vi "thermistor_manager_2.vi"(8 "ready for output (T)":bool=TRUE, 9 "input valid":bool=TRUE, 11 "indexed_voltage":T2) -> (3 "indexed_temperature":T1)   [LabVIEW 2018]
uses:
  indexed_analog.ctl
  indexed_fxp32_16.ctl
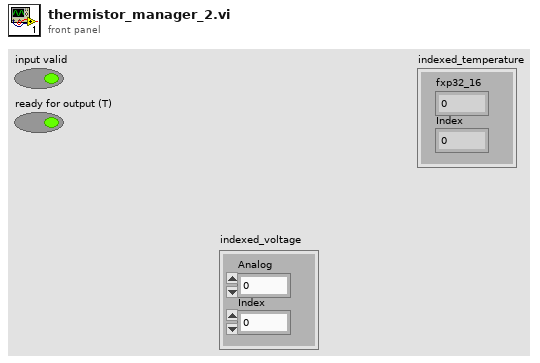
[diagram p1: front panel]
types:
  T1 = typedef "indexed_fxp32_16.ctl" = cluster{"fxp32_16":fxp<+/-,32,16>, "Index":fxp<+,3,3>}
  T2 = typedef "indexed_analog.ctl" = cluster{"Analog":fxp<+/-,24,5>, "Index":fxp<+,3,3>}
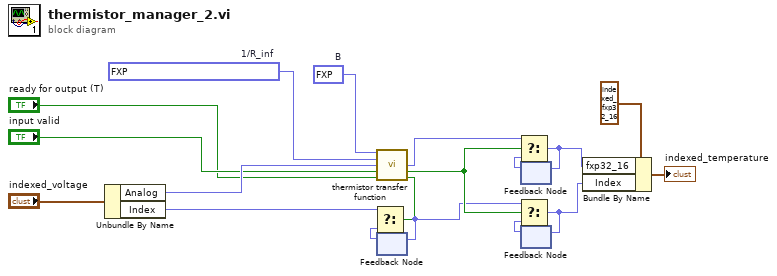
[diagram p0: block diagram]
diagram:
  w16 = fxp<+,32,7> 10.047783523797989  # 1/R_inf
  w17 = fxp<+/-,32,16> 3434.0  # B
  n1 = Unbundle By Name("indexed_voltage") -> ("Analog"=w14:fxp<+/-,24,5>, "Index"=w2:fxp<+,3,3>)
  n2 = call "thermistor transfer function.vi"("B"=w17, "1/R_inf"=w16, "V"=w14, "input valid"="input valid", "ready for output (T)"="ready for output (T)") -> ("Temperature"=w7:fxp<+/-,32,16>, "output valid"=w9:bool, "ready for input"=w15:bool)  [unwired: 8 in]
  n3 = feedback #1() -> (w1:fxp<+,3,3>)  [unwired: 1 in]
  n4 = Select(t=w2, s=w15, f=w1) -> (s? t:f=w8:fxp<+,3,3>)
  n5 = feedback-in #1(w8) -> ()
  n6 = feedback #2() -> (w10:fxp<+/-,32,16>)  [unwired: 1 in]
  n7 = Select(t=w7, s=w9, f=w10) -> (s? t:f=w6:fxp<+/-,32,16>)
  n8 = feedback-in #2(w6) -> ()
  n9 = feedback #3() -> (w11:fxp<+,3,3>)  [unwired: 1 in]
  n10 = Select(t=w8, s=w9, f=w11) -> (s? t:f=w3:fxp<+,3,3>)
  n11 = feedback-in #3(w3) -> ()
  n12 = Bundle By Name(cluster=T1 {"fxp32_16"=0.0, "Index"=0.0} ("indexed_analog"), "fxp32_16"=w6, "Index"=w3) -> (→"indexed_temperature":T1)
